vi "AOTF_Analog_Pulse_Switch.vi"(6 "Array 2":dbl[][](array[numeric]), 7 "Number of active lines":u8, 9 "AOTF-Digital switch in":tag="/Dev1/PFI1", 10 "Pictures per pixel":u8, 11 "Pulse per Wavelength":u8[](array[numeric])) -> (0 "error out":errorcluster, 3 "task out":refnum<k21>)   [LabVIEW 2011]
uses:
  <vilib>/DAQmx/write.llb/DAQmx Write (Analog 2D DBL NChan NSamp).vi
  <vilib>/DAQmx/configure/timing.llb/DAQmx Timing (Sample Clock).vi
  <vilib>/DAQmx/miscellaneous.llb/DAQmx Fill In Error Info.vi
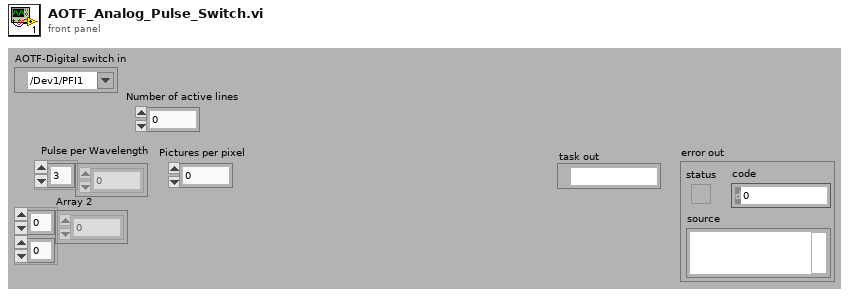
[diagram p1: front panel]
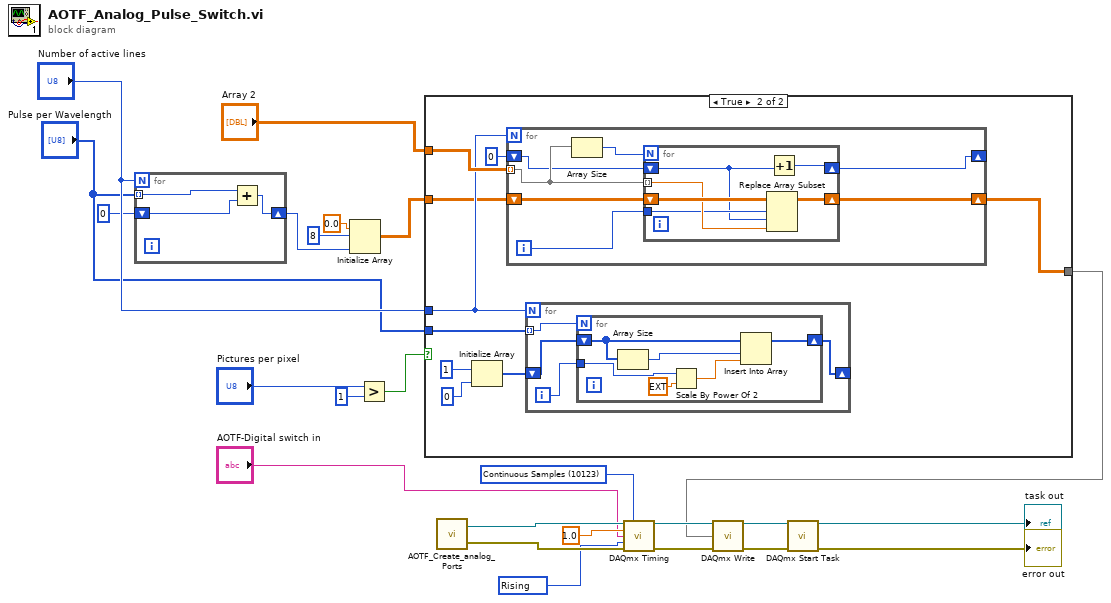
[diagram p0: block diagram]
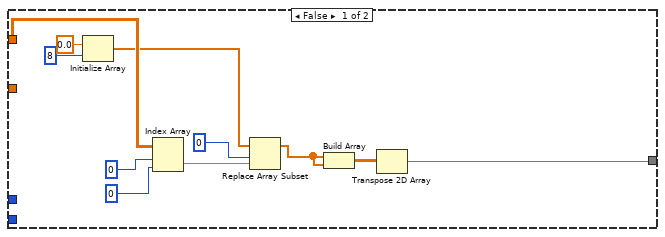
[diagram p2: hidden frame]
diagram:
  w21 = 10123 items=["Finite Samples"=10178, "Continuous Samples"=10123, "Hardware Timed Single Point"=12522] ("sample mode")
  w12 = 10280 items=["Rising"=10280, "Falling"=10171] ("active edge")
  n1 = for {
    N: "Number of active lines" -> [_]
    tunnel: "Pulse per Wavelength" -> [w25] mode=indexing
    shift-right: [w27] -> w3
    shift-left: 0 -> [w26]
    n2 = Add(x=w25, y=w26) -> (x+y=w27:i32)
  }
  n3 = Initialize Array(0.0 ("element"), 8 ("dimension size"), w3) -> (w6:dbl[][])
  n4 = Greater?(x="Pictures per pixel", y=u8 1) -> (0:w22:bool)
  n5 = case shown="True" w22 {
    tunnel: "Number of active lines" -> [_ w42]
    tunnel: "Pulse per Wavelength" -> [_ w47]
    tunnel: "Array 2" -> [w36 w43]
    tunnel: [w32 w40] -> w9
    tunnel: w6 -> [_ w41]
    frame False {
      n6 = Initialize Array(0.0 ("element"), 8 ("dimension size")) -> (w28:dbl[])
      n7 = Index Array(array=w36, index (row)=0, index (col)=0 ("disabled index (col)")) -> (element=w35:dbl)
      n8 = Replace Array Subset(array=w28, new element=w35, index=0) -> (w31:dbl[])
      n9 = Build Array(w31, w31) -> (w33:dbl[][])
      n10 = Transpose 2D Array(2D array=w33) -> (transposed array=w32:dbl[][])
    }
    frame True {
      n11 = Initialize Array(1 ("element"), 0 ("dimension size")) -> (w46:i32[])
      n12 = for {
        N: w42 -> [_]
        tunnel: w43 -> [w51] mode=indexing
        shift-right: [w53] -> w40
        shift-left: w41 -> [w54]
        shift-right: [w49] -> _
        shift-left: 0 -> [w48]
        i -> [w52]
        n13 = Array Size(array=w51) -> (size(s)=w50:i32)
        n14 = for {
          N: w50 -> [_]
          shift-right: [w59] -> w53
          shift-left: w54 -> [w60]
          tunnel: w51 -> [w58] mode=indexing
          tunnel: w52 -> [w57]
          shift-right: [w56] -> w49
          shift-left: w48 -> [w55]
          n15 = Replace Array Subset(array=w60, new element=w58, index (row)=w57, index (col)=w55) -> (w59:dbl[][])
          n16 = Increment(x=w55) -> (x+1=w56:i32)
        }
      }
      n17 = for {
        N: w42 -> [_]
        tunnel: w47 -> [w64] mode=indexing
        shift-right: [w62] -> _
        shift-left: w46 -> [w63]
        i -> [w61]
        n18 = for {
          N: w64 -> [_]
          shift-right: [w70] -> w62
          shift-left: w63 -> [w69]
          tunnel: w61 -> [w66]
          n19 = Array Size(array=w69) -> (size(s)=w68:i32)
          n20 = Scale By Power Of 2(n=w66, x=ext 1.0) -> (x*2^n=w67:ext)
          n21 = Insert Into Array(array=w69, index=w68, new element=w67) -> (w70:i32[])
        }
      }
    }
  }
  n22 = call "AOTF_Create_analog_Ports.vi"() -> ("task out"=w20:refnum<k21>, "error out"=w19:errorcluster)  [unwired: 1 in]
  n23 = call-poly <vilib>:"DAQmx Timing.vi"("task/channels in"=w20, "sample mode"=w21, "rate"=1.0, "source"="AOTF-Digital switch in", "active edge"=w12, "error in"=w19) -> ("task out"=w18:refnum<k21>, "error out"=w17:errorcluster)  [unwired: 1 in, 7 out]
  n24 = call-poly <vilib>:"DAQmx Write.vi"("task/channels in"=w18, "data"=w9, "error in"=w17) -> ("task out"=w16:refnum<k21>, "error out"=w15:errorcluster)  [unwired: 1 in, 10 out]
  n25 = call <vilib>:"DAQmx Start Task.vi"("task/channels in"=w16, "error in"=w15) -> ("task out"=→"task out":refnum<k21>, "error out"=→"error out":errorcluster)  [unwired: 12 out]
